vi "Init.vi"(8 "error in":errorcluster, 11 "NEO480 in":refnum<class "Virtual Thermometer.lvclass">) -> (0 "error out":errorcluster, 3 "NEO480 out":refnum<class "Virtual Thermometer.lvclass">)   [LabVIEW 2024, in "Virtual Thermometer.lvclass"]
uses:
  Virtual Thermometer.lvclass
  Virtual Thermometer.lvclass/Virtual Thermometer.ctl
  Interfaces/IConfiguration/IConfiguration.lvclass
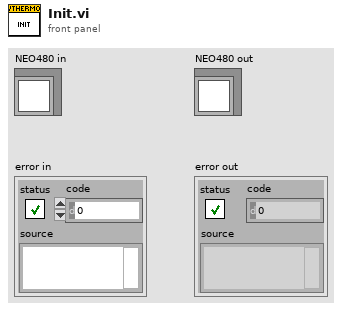
[diagram p1: front panel]
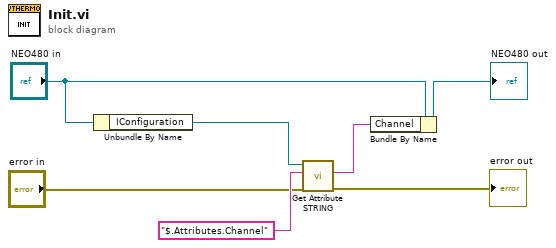
[diagram p0: block diagram]
diagram:
  n1 = Unbundle By Name("NEO480 in") -> ("IConfiguration"=w7:refnum<class "IConfiguration.lvclass">)
  n2 = call-dynamic "Get Attribute STRING.vi"("error in"="error in", "Attribute"="$.Attributes.Channel", "IConfiguration in"=w7) -> ("error out"=→"error out":errorcluster, "Value"=w1:string)  [unwired: 6 in, 1 out]
  n3 = Bundle By Name(cluster="NEO480 in", "Channel"=w1) -> (→"NEO480 out":refnum<class "Virtual Thermometer.lvclass">)
